vi "TestFilter.vi"(0 "Image In":T2, 1 "Red BCG Values (Brightness 1)":T1={"Brightness"=142.42021, "Contrast"=69.80851, "Gamma"=2.51808}, 2 "Green BCG Values (Brightness 1)":T1={"Brightness"=142.42021, "Contrast"=69.80851, "Gamma"=2.51808}, 3 "Blue BCG Values (Brightness 1)":T1={"Brightness"=142.42021, "Contrast"=69.80851, "Gamma"=2.51808}, 4 "Range (Threshold 1)":cluster{"Lower value":sgl, "Upper value":sgl}={"Lower value"=109.28571, "Upper value"=255.0}, 7 "error in":errorcluster) -> (20 "Image Out":T2, 27 "error out":errorcluster)   [LabVIEW 2020]
uses:
  <vilib>/vision/Image Controls.llb/IMAQ Image.ctl
  <vilib>/vision/NI_Vision_Development_Module.lvlib
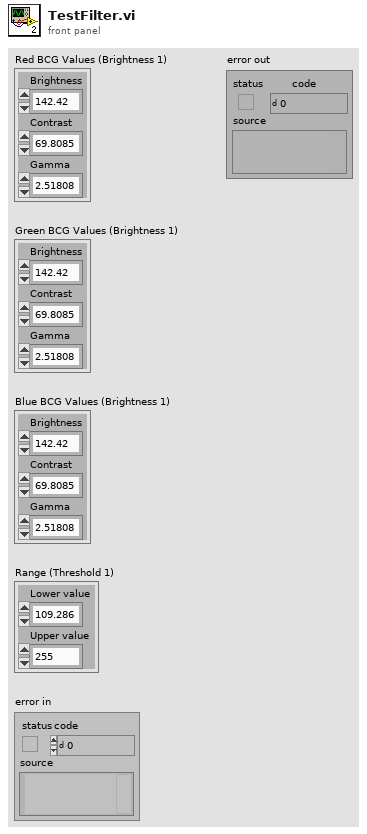
[diagram p1: front panel]
types:
  T1 = cluster{"Brightness":sgl, "Contrast":sgl, "Gamma":sgl}
  T2 = typedef "IMAQ Image.ctl" = refnum<image>
  T3 = cluster{"Measurement Parameter":i32, "Range Lower Value":dbl, "Range Upper Value":dbl, "Range":bool, "Measurement Type":bool}[]
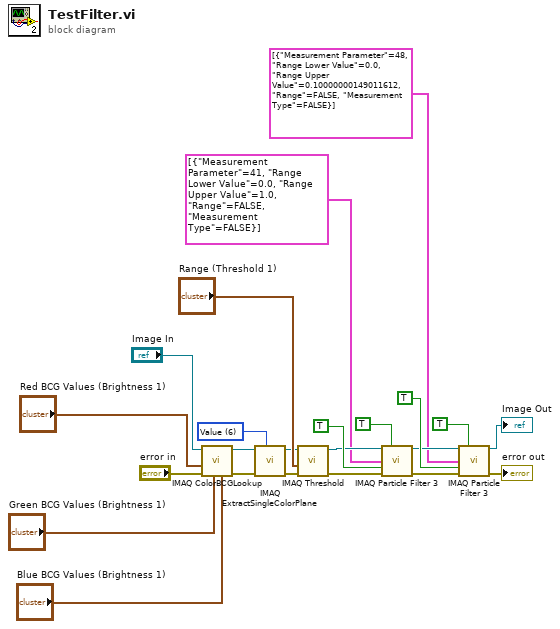
[diagram p0: block diagram]
diagram:
  w18 = 6 items=["Red", "Green", "Blue", "Hue", "Saturation", "Luminance", "Value", "Intensity"] ("Color Plane")
  n1 = call "IMAQ ColorBCGLookup"("Blue BCG Values"="Blue BCG Values (Brightness 1)", "Green BCG Values"="Green BCG Values (Brightness 1)", "error in (no error)"="error in", "Red BCG Values"="Red BCG Values (Brightness 1)", "Image Src"="Image In") -> ("error out"=w16:errorcluster, "Image Dst Out"=w17:T2)  [unwired: 2 in, 3 out]
  n2 = call "IMAQ ExtractSingleColorPlane"("Color Plane"=w18, "error in (no error)"=w16, "Image Src"=w17) -> ("error out"=w13:errorcluster, "Image Dst Out"=w14:T2)  [unwired: 1 in, 6 out]
  n3 = call "IMAQ Threshold"("error in (no error)"=w13, "Range"="Range (Threshold 1)", "Image Src"=w14) -> ("error out"=w9:errorcluster, "Image Dst Out"=w10:T2)  [unwired: 3 in, 4 out]
  n4 = call "IMAQ Particle Filter 3"("Image Src"=w10, "Connectivity 4/8 (8)"=TRUE, "Selection Values"=T3 [{"Measurement Parameter"=41, "Range Lower Value"=0.0, "Range Upper Value"=1.0, "Range"=FALSE, "Measurement Type"=FALSE}], "Keep/Remove Particles (F)"=TRUE ("Keep/Remove Particles"), "error in (no error)"=w9) -> ("Image Dst Out"=w3:T2, "error out"=w2:errorcluster)  [unwired: 4 in, 5 out]
  n5 = call "IMAQ Particle Filter 3"("Image Src"=w3, "Connectivity 4/8 (8)"=TRUE, "Selection Values"=T3 [{"Measurement Parameter"=48, "Range Lower Value"=0.0, "Range Upper Value"=0.10000000149011612, "Range"=FALSE, "Measurement Type"=FALSE}], "Keep/Remove Particles (F)"=TRUE ("Keep/Remove Particles"), "error in (no error)"=w2) -> ("Image Dst Out"=→"Image Out":T2, "error out"=→"error out":errorcluster)  [unwired: 4 in, 5 out]
